vi "Stop.vi"(8 "error in (no error)":errorcluster, 11 "Analog Output in":refnum<class "Analog output.lvclass">) -> (0 "error out":errorcluster, 3 "connection ID":i32)   [LabVIEW 2009, in "MicroDAQ.lvlib" / "Analog output.lvclass"]
doc: "Stops generation, drops output to 0."
uses:
  <instrlib>/MicroDAQ/Channel/Analog Output/Analog output.lvclass
  <instrlib>/MicroDAQ/Channel/Analog Output/Analog output.lvclass/Analog output.ctl
  <instrlib>/MicroDAQ/Channel/Channel.lvclass
  <instrlib>/MicroDAQ/Mlink library wraper/mlink.lvlib
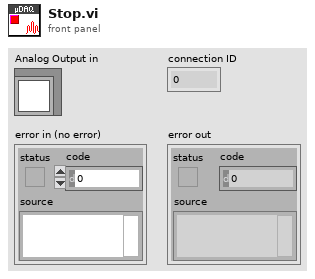
[diagram p1: front panel]
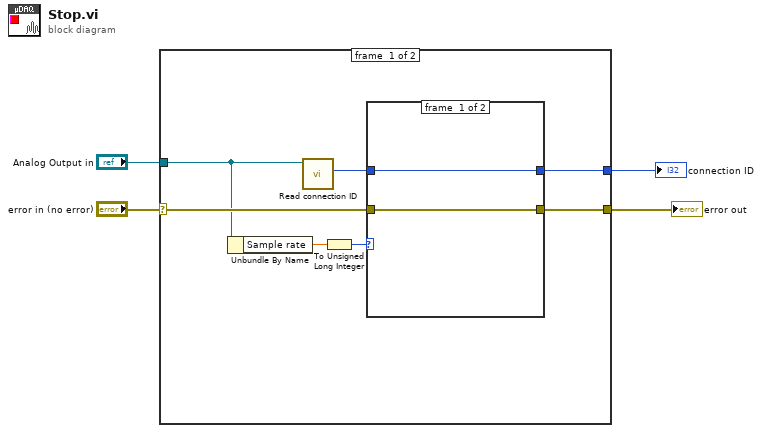
[diagram p0: block diagram]
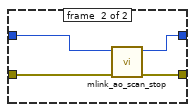
[diagram p2: hidden frame]
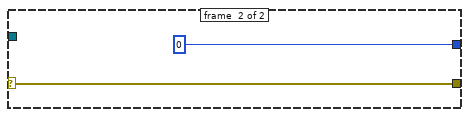
[diagram p3: hidden frame]
diagram:
  n1 = case shown="No Error" "error in (no error)" {
    selector: "error in (no error)" -> [w10 w19]
    tunnel: "Analog Output in" -> [w7 _]
    tunnel: [w11 w19] -> w3
    tunnel: [w9 0 ("connection ID out")] -> w1
    frame #0 {
      n2 = Unbundle By Name(w7) -> ("Sample rate"=w8:dbl)
      n3 = call <instrlib>:"Read connection ID.vi"("Task in"=w7) -> ("connection ID"=w6:i32)  [unwired: 9 in, 1 out]
      n4 = To Unsigned Long Integer(number=w8) -> (unsigned 32bit integer=w5:u32)
      n5 = case shown="Default" w5 {
        tunnel: [w12 w17] -> w11
        tunnel: w10 -> [w12 w16]
        tunnel: [w13 w15] -> w9
        tunnel: w6 -> [w13 w14]
        frame #0 {
        }
        frame #1 {
          n6 = call <instrlib>:"mlink_ao_scan_stop.vi"("error in (no error)"=w16, "connection ID"=w14) -> ("error out"=w17:errorcluster, "connection ID out"=w15:i32)  [unwired: 8 in]
        }
      }
    }
    frame #1 {
    }
  }
  "error out" <- w3
  "connection ID" <- w1
